vi "Begin.vi"(8 "error in":errorcluster) -> (0 "error out":errorcluster)   [LabVIEW 2020]
doc: "Called before other user functions, this VI is expected to open initial I/O refnums, load in file data, and do all program initialization. Notice that the <B>error out</B> terminal is simply used for data flow. Wiring it to other structures or subVIs ensures that this VI runs first."
uses:
  <vilib>/Rock Robotics/WPI/DriverStation/WPI_DriverStationRobotMode2.ctl
  <vilib>/Rock Robotics/WPI/Joystick/WPI_JoystickDeviceEnum.ctl
  <vilib>/Rock Robotics/SystemInterfaces/i2clib/i2c_bus.ctl
  <vilib>/Rock Robotics/WPI/Solenoid/WPI_SolenoidChannel.ctl
  <vilib>/Rock Robotics/SystemInterfaces/DIO/FPGA_DIOChannel.ctl
  Robot Global Data.vi
  <vilib>/Rock Robotics/Network Tables/NT Write String Array.vi
  <vilib>/Rock Robotics/WPI/ThirdParty/Phoenix-LabVIEW/Motor Controller/Get/CTRE_Phoenix_MotorController_GetSelectedSensorData.vi
  <vilib>/Rock Robotics/WPI/Solenoid/WPI_SolenoidOpenDouble.vi
  <vilib>/Rock Robotics/WPI/Switch/WPI_SwitchOpenLimit.vi
  <vilib>/Rock Robotics/WPI/Switch/WPI_SwitchOpenCounting.vi
  <vilib>/Rock Robotics/WPI/ThirdParty/Phoenix-LabVIEW/Motor Controller/Get/CTRE_Phoenix_MotorController_IntegratedSensorData_TalonFX.vi
  GlobalAutonVariables.vi
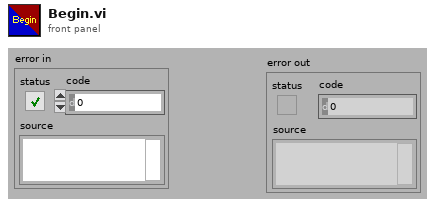
[diagram p1: front panel]
types:
  T1 = typedef "FPGA_DIOChannel.ctl" = enum8{"DIO 0", "DIO 1", "DIO 2", "DIO 3", "DIO 4", "DIO 5", "DIO 6", "DIO 7", "DIO 8", "DIO 9", "DIO MXP 0", "DIO MXP 1", "DIO MXP 2", "DIO MXP 3", "DIO MXP 4", "DIO MXP 5", "DIO MXP 6", "DIO MXP 7", "DIO MXP 8", "DIO MXP 9", "DIO MXP 10", "DIO MXP 11", "DIO MXP 12", "DIO MXP 13", "DIO MXP 14", "DIO MXP 15", "SPI Port CS1", "SPI Port CS2", "SPI Port CS3", "SPI Port MISO", "SPI Port MOSI", "Invalid"}
  T2 = typedef "WPI_SolenoidChannel.ctl" = enum8{"Solenoid 0", "Solenoid 1", "Solenoid 2", "Solenoid 3", "Solenoid 4", "Solenoid 5", "Solenoid 6", "Solenoid 7", "Solenoid 8", "Solenoid 9", "Solenoid 10", "Solenoid 11", "Solenoid 12", "Solenoid 13", "Solenoid 14", "Solenoid 15", "Invalid"}
  T3 = typedef "i2c_bus.ctl" = enum16{"I2C On-Board", "I2C MXP", "Invalid"}
  T4 = typedef "WPI_JoystickDeviceEnum.ctl" = enum16{"USB 0", "USB 1", "USB 2", "USB 3", "USB 4", "USB 5"}
  T5 = typedef "WPI_DriverStationRobotMode2.ctl" = enum16{"Autonomous Disabled", "Autonomous Enabled", "Teleop Disabled", "Teleop Enabled", "Disconnected", "Finish", "Test Disabled", "Test Enabled", "Emergency Stopped"}
  T6 = typedef "WPI_CompressorDevRef.ctl" = cluster{"DevStatus":errorcluster, "Pneumatics Control Module":u8}
  T7 = typedef "WPI_SolenoidDevRef.ctl" = cluster{"DevStatus":errorcluster, "Pneumatics Control Module":u8, "Forward Solenoid Channel":T2, "Reverse Solenoid Channel":T2}
  T8 = typedef "WPI_JoystickDevRef.ctl" = cluster{"Device":T4}
  T9 = typedef "WPI_MotorControlDeviceRef.ctl" = cluster{"DeviceStatus":errorcluster, "Type":T10, "PWM":cluster{"PWM Channel":T11, "DeadBand":T12}, "CAN":cluster{"Device Number":u8, "SetOutput VI Ref":variant, "GetOutput VI Ref":variant, "Enable VI Ref":variant, "Disable VI Ref":variant, "Data":variant}, "Invert":bool, "DIO PWM":cluster{"PWM \"Enable\" Channel":T11, "DIOChannel":T1, "PWM Rate":dbl}}
  T10 = typedef "WPI_MotorControlType.ctl" = enum16{"PWM", "CAN", "DIO PWM"}
  T11 = typedef "FPGA_DIOPWMChannel.ctl" = enum8{"PWM 0", "PWM 1", "PWM 2", "PWM 3", "PWM 4", "PWM 5", "PWM 6", "PWM 7", "PWM 8", "PWM 9", "PWM MXP 0", "PWM MXP 1", "PWM MXP 2", "PWM MXP 3", "PWM MXP 4", "PWM MXP 5", "PWM MXP 6", "PWM MXP 7", "PWM MXP 8", "PWM MXP 9", "Invalid"}
  T12 = typedef "WPI_PWMDeadband.ctl" = cluster{"Name":string, "maxPositivePwm":i32, "minPositivePwm":i32, "centerPwm":i32, "maxNegativePwm":i32, "minNegativePwm":i32, "angularRange":u16}
  T13 = typedef "Color Sensor V3 DevRef.ctl" = cluster{"I2CDevRef":T14}
  T14 = typedef "WPI_I2CDevRef.ctl" = cluster{"DevStatus":errorcluster, "Device Address":u8, "Handle":i32, "I2C Bus":T3}
  T15 = typedef "CTRE_PigeonIMU_DeviceRef.ctl" = cluster{"DeviceStatus":errorcluster, "Device Number":u8, "Type":T16, "Device ID":u32, "Handle":u64, "UsageFrame":u32, "Library Path":path}
  T16 = typedef "CTRE_PigeonIMU_ConnectionType.ctl" = u32
  T17 = typedef "CTRE_Phoenix_CANcoder_DeviceRef.ctl" = cluster{"DeviceStatus":errorcluster, "Device Number":u8, "Handle":u64, "UsageFrame":u32, "Library Path":path}
  T18 = typedef "WPI_SwitchDevRef.ctl" = cluster{"DevStatus":errorcluster, "DIO Channel":T1, "CntIndex":T19, "Normally Closed":bool}
  T19 = typedef "FPGA_CounterCtrSystemIndex.ctl" = enum8{"Ctr 0", "Ctr 1", "Ctr 2", "Ctr 3", "Ctr 4", "Ctr 5", "Ctr 6", "Ctr 7", "Invalid"}
  T20 = enum16{"open", "replace", "create", "open or create", "replace or create", "replace or create with confirmation"}
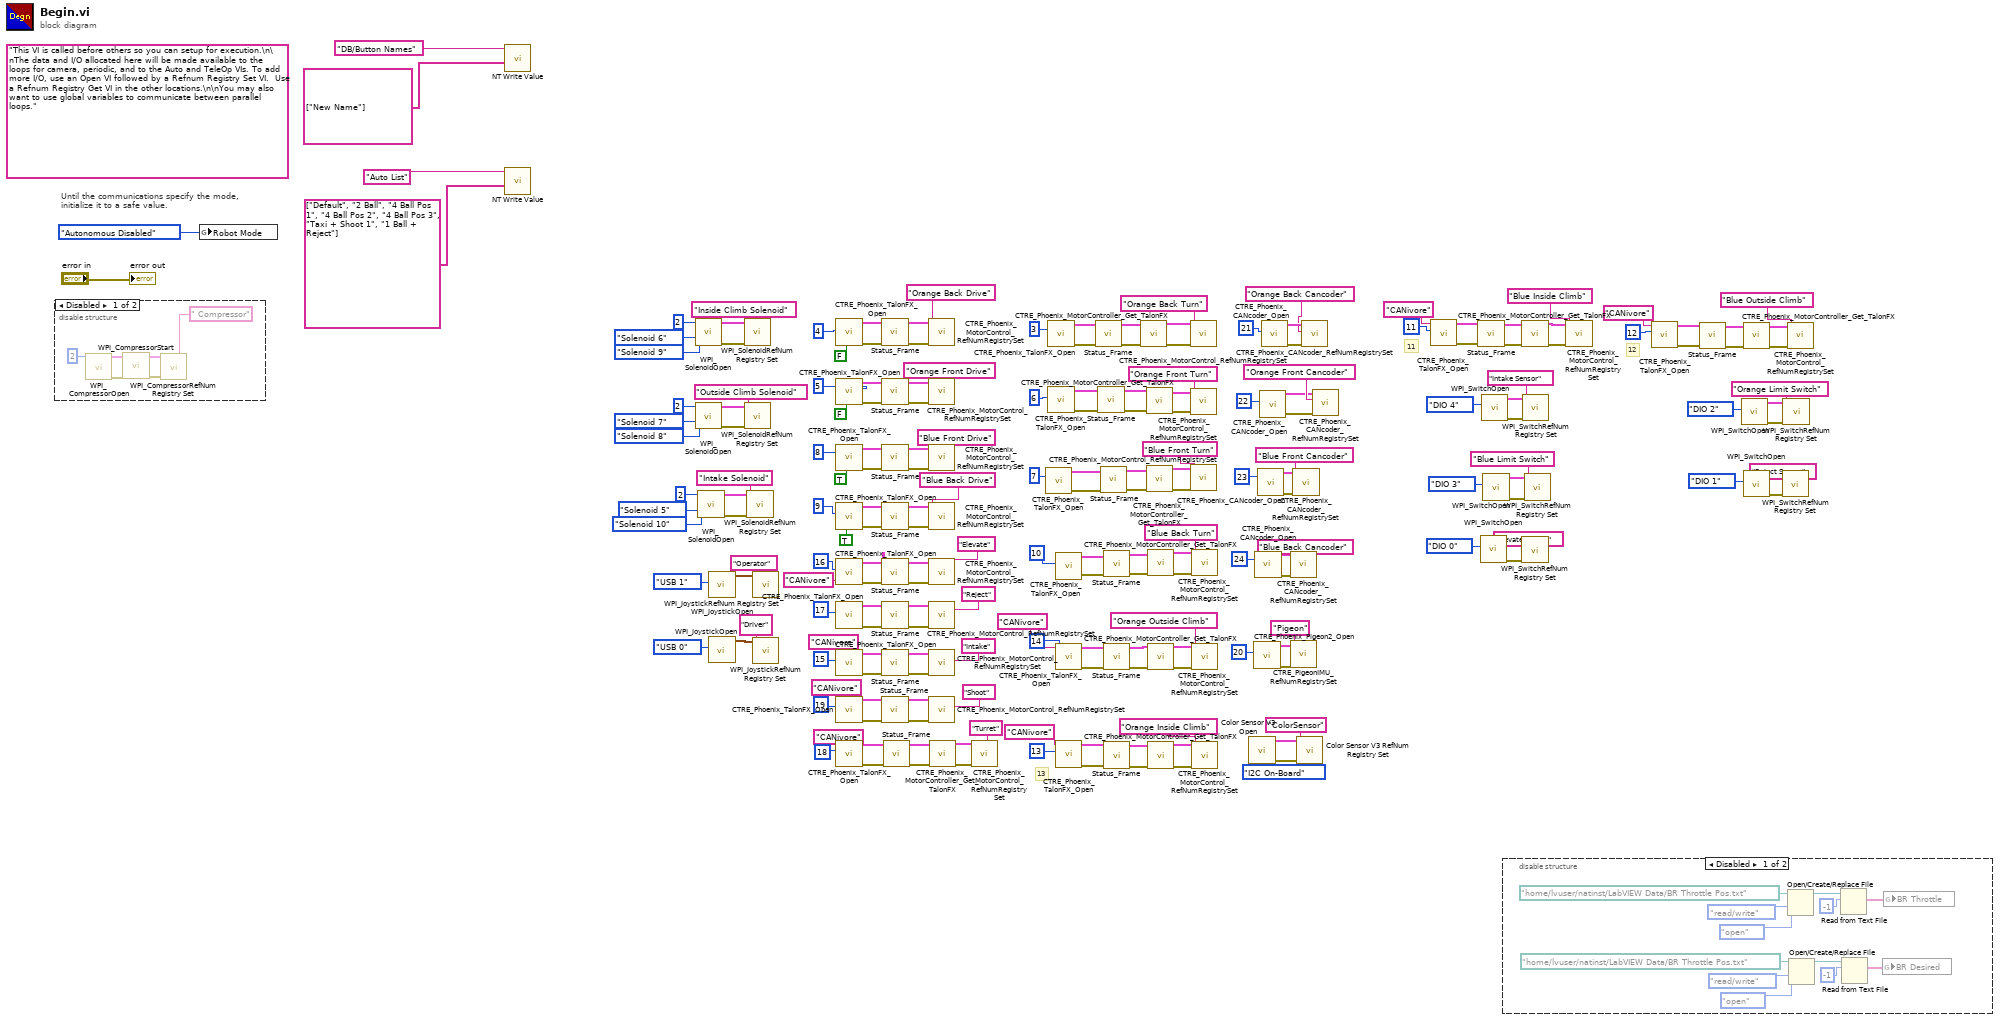
[diagram p0: block diagram]
diagram:
  (unwired) "This VI is called before others so you can setup for execution.\n\nThe data and I/O allocated here will be made available to the loops for camera, periodic, and to the Auto and TeleOp VIs. To add more I/O, use an Open VI followed by a Refnum Registry Set VI.  Use a Refnum Registry Get VI in the other locations.\n\nYou may also want to use global variables to communicate between parallel loops."
  # "13"
  # "12"
  # "11"
  # "Until the communications specify the mode,\ninitialize it to a safe value."
  n1 = disable-structure shown="Disabled" {
    frame Disabled {
      n2 = call <vilib>:"WPI_CompressorOpen.vi"("Pneumatics device (def)"=u8 2) -> ("CompressorDevRef"=w211:T6, "error out"=w212:errorcluster)  [unwired: 13 in]
      n3 = call <vilib>:"WPI_CompressorStart.vi"("error in (no error)"=w212, "CompressorDevRef"=w211) -> ("error out"=w210:errorcluster, "CompressorDevRef"=w209:T6)  [unwired: 8 in]
      n4 = call <vilib>:"WPI_CompressorRefNum Registry Set.vi"("error in (no error)"=w210, "refnum name"=" Compressor", "CompressorDevRef"=w209) -> ()  [unwired: 7 in, 2 out]
    }
    frame Enabled {
    }
  }
  n5 = global write "Robot Global Data.vi" "Robot Mode"(WPI_DriverStationRobotMode2."Autonomous Disabled" ("Robot Mode")) -> ()
  n6 = call-poly <vilib>:"NT Write Value.vi"("String Array"=string[] ["New Name"], "Name"="DB/Button Names") -> ()  [unwired: 9 in, 1 out]
  n7 = call-poly <vilib>:"NT Write Value.vi"("String Array"=string[] ["Default", "2 Ball", "4 Ball Pos 1", "4 Ball Pos 2", "4 Ball Pos 3", "Taxi + Shoot 1", "1 Ball + Reject"], "Name"="Auto List") -> ()  [unwired: 9 in, 1 out]
  n8 = call-poly <vilib>:"WPI_SolenoidOpen.vi"("Reverse Solenoid Channel"=WPI_SolenoidChannel."Solenoid 9", "Forward Solenoid Channel"=WPI_SolenoidChannel."Solenoid 6", "Pneumatics Device (def)"=u8 2) -> ("error out"=w155:errorcluster, "SolenoidDevRef"=w154:T7)  [unwired: 7 in]
  n9 = call-poly <vilib>:"WPI_SolenoidOpen.vi"("Reverse Solenoid Channel"=WPI_SolenoidChannel."Solenoid 8", "Forward Solenoid Channel"=WPI_SolenoidChannel."Solenoid 7", "Pneumatics Device (def)"=u8 2) -> ("error out"=w152:errorcluster, "SolenoidDevRef"=w151:T7)  [unwired: 7 in]
  n10 = call-poly <vilib>:"WPI_SolenoidOpen.vi"("Reverse Solenoid Channel"=WPI_SolenoidChannel."Solenoid 10", "Forward Solenoid Channel"=WPI_SolenoidChannel."Solenoid 5", "Pneumatics Device (def)"=u8 2) -> ("error out"=w149:errorcluster, "SolenoidDevRef"=w148:T7)  [unwired: 7 in]
  n11 = call <vilib>:"WPI_JoystickOpen.vi"("JoystickDevice"=WPI_JoystickDeviceEnum."USB 1") -> ("JoystickDevRef"=w196:T8)  [unwired: 10 in]
  n12 = call <vilib>:"WPI_JoystickOpen.vi"("JoystickDevice"=WPI_JoystickDeviceEnum."USB 0") -> ("JoystickDevRef"=w204:T8)  [unwired: 10 in]
  n13 = call <vilib>:"WPI_SolenoidRefNum Registry Set.vi"("error in (no error)"=w155, "refnum name"="Inside Climb Solenoid", "SolenoidDevRef"=w154) -> ()  [unwired: 7 in, 2 out]
  n14 = call <vilib>:"WPI_SolenoidRefNum Registry Set.vi"("error in (no error)"=w152, "refnum name"="Outside Climb Solenoid", "SolenoidDevRef"=w151) -> ()  [unwired: 7 in, 2 out]
  n15 = call <vilib>:"WPI_SolenoidRefNum Registry Set.vi"("error in (no error)"=w149, "refnum name"="Intake Solenoid", "SolenoidDevRef"=w148) -> ()  [unwired: 7 in, 2 out]
  n16 = call <vilib>:"WPI_JoystickRefNum Registry Set.vi"("refnum name"="Operator", "JoystickDevRef"=w196) -> ()  [unwired: 8 in, 2 out]
  n17 = call <vilib>:"WPI_JoystickRefNum Registry Set.vi"("refnum name"="Driver", "JoystickDevRef"=w204) -> ()  [unwired: 8 in, 2 out]
  n18 = call <vilib>:"CTRE_Phoenix_TalonFX_Open.vi"("Invert"=FALSE, "Device Number"=u8 4) -> ("error out"=w75:errorcluster, "PhoenixMotorControlDevRef"=w76:T9)  [unwired: 8 in]
  n19 = call <vilib>:"CTRE_Phoenix_TalonFX_Open.vi"("Invert"=FALSE, "Device Number"=u8 5) -> ("error out"=w68:errorcluster, "PhoenixMotorControlDevRef"=w67:T9)  [unwired: 8 in]
  n20 = call <vilib>:"CTRE_Phoenix_TalonFX_Open.vi"("Invert"=TRUE, "Device Number"=u8 8) -> ("error out"=w72:errorcluster, "PhoenixMotorControlDevRef"=w69:T9)  [unwired: 8 in]
  n21 = call <vilib>:"CTRE_Phoenix_TalonFX_Open.vi"("Invert"=TRUE, "Device Number"=u8 9) -> ("error out"=w61:errorcluster, "PhoenixMotorControlDevRef"=w64:T9)  [unwired: 8 in]
  n22 = call <vilib>:"CTRE_Phoenix_TalonFX_Open.vi"("Device Number"=u8 16, "CAN Bus"="CANivore") -> ("error out"=w57:errorcluster, "PhoenixMotorControlDevRef"=w60:T9)  [unwired: 8 in]
  n23 = call <vilib>:"CTRE_Phoenix_TalonFX_Open.vi"("Device Number"=u8 17) -> ("error out"=w53:errorcluster, "PhoenixMotorControlDevRef"=w56:T9)  [unwired: 9 in]
  n24 = call <vilib>:"CTRE_Phoenix_TalonFX_Open.vi"("Device Number"=u8 15, "CAN Bus"="CANivore") -> ("error out"=w49:errorcluster, "PhoenixMotorControlDevRef"=w52:T9)  [unwired: 8 in]
  n25 = call <vilib>:"CTRE_Phoenix_TalonFX_Open.vi"("Device Number"=u8 19, "CAN Bus"="CANivore") -> ("error out"=w45:errorcluster, "PhoenixMotorControlDevRef"=w48:T9)  [unwired: 8 in]
  n26 = call <vilib>:"CTRE_Phoenix_TalonFX_Open.vi"("Device Number"=u8 18, "CAN Bus"="CANivore") -> ("error out"=w42:errorcluster, "PhoenixMotorControlDevRef"=w43:T9)  [unwired: 8 in]
  n27 = call "Status_Frame.vi"("error in (no error)"=w75, "Motor Control DevRef"=w76) -> ("error out"=w74:errorcluster, "PhoenixMotorControlDevRef"=w73:T9)  [unwired: 8 in]
  n28 = call "Status_Frame.vi"("error in (no error)"=w68, "Motor Control DevRef"=w67) -> ("error out"=w65:errorcluster, "PhoenixMotorControlDevRef"=w66:T9)  [unwired: 8 in]
  n29 = call "Status_Frame.vi"("error in (no error)"=w72, "Motor Control DevRef"=w69) -> ("error out"=w71:errorcluster, "PhoenixMotorControlDevRef"=w70:T9)  [unwired: 8 in]
  n30 = call "Status_Frame.vi"("error in (no error)"=w61, "Motor Control DevRef"=w64) -> ("error out"=w62:errorcluster, "PhoenixMotorControlDevRef"=w63:T9)  [unwired: 8 in]
  n31 = call "Status_Frame.vi"("error in (no error)"=w57, "Motor Control DevRef"=w60) -> ("error out"=w58:errorcluster, "PhoenixMotorControlDevRef"=w59:T9)  [unwired: 8 in]
  n32 = call "Status_Frame.vi"("error in (no error)"=w53, "Motor Control DevRef"=w56) -> ("error out"=w54:errorcluster, "PhoenixMotorControlDevRef"=w55:T9)  [unwired: 8 in]
  n33 = call "Status_Frame.vi"("error in (no error)"=w49, "Motor Control DevRef"=w52) -> ("error out"=w50:errorcluster, "PhoenixMotorControlDevRef"=w51:T9)  [unwired: 8 in]
  n34 = call "Status_Frame.vi"("error in (no error)"=w45, "Motor Control DevRef"=w48) -> ("error out"=w46:errorcluster, "PhoenixMotorControlDevRef"=w47:T9)  [unwired: 8 in]
  n35 = call "Status_Frame.vi"("error in (no error)"=w42, "Motor Control DevRef"=w43) -> ("error out"=w3:errorcluster, "PhoenixMotorControlDevRef"=w4:T9)  [unwired: 8 in]
  n36 = call <vilib>:"CTRE_Phoenix_MotorControl_RefNumRegistrySet.vi"("error in (no error)"=w74, "refnum name"="Orange Back Drive", "PhoenixMotorControlDevRef"=w73) -> ()  [unwired: 7 in, 2 out]
  n37 = call <vilib>:"CTRE_Phoenix_MotorControl_RefNumRegistrySet.vi"("error in (no error)"=w65, "refnum name"="Orange Front Drive", "PhoenixMotorControlDevRef"=w66) -> ()  [unwired: 7 in, 2 out]
  n38 = call <vilib>:"CTRE_Phoenix_MotorControl_RefNumRegistrySet.vi"("error in (no error)"=w71, "refnum name"="Blue Front Drive", "PhoenixMotorControlDevRef"=w70) -> ()  [unwired: 7 in, 2 out]
  n39 = call <vilib>:"CTRE_Phoenix_MotorControl_RefNumRegistrySet.vi"("error in (no error)"=w62, "refnum name"="Blue Back Drive", "PhoenixMotorControlDevRef"=w63) -> ()  [unwired: 7 in, 2 out]
  n40 = call <vilib>:"CTRE_Phoenix_MotorControl_RefNumRegistrySet.vi"("error in (no error)"=w58, "refnum name"="Elevate", "PhoenixMotorControlDevRef"=w59) -> ()  [unwired: 7 in, 2 out]
  n41 = call <vilib>:"CTRE_Phoenix_MotorControl_RefNumRegistrySet.vi"("error in (no error)"=w54, "refnum name"="Reject", "PhoenixMotorControlDevRef"=w55) -> ()  [unwired: 7 in, 2 out]
  n42 = call <vilib>:"CTRE_Phoenix_MotorControl_RefNumRegistrySet.vi"("error in (no error)"=w50, "refnum name"="Intake", "PhoenixMotorControlDevRef"=w51) -> ()  [unwired: 7 in, 2 out]
  n43 = call <vilib>:"CTRE_Phoenix_MotorControl_RefNumRegistrySet.vi"("error in (no error)"=w46, "refnum name"="Shoot", "PhoenixMotorControlDevRef"=w47) -> ()  [unwired: 7 in, 2 out]
  n44 = call-poly <vilib>:"CTRE_Phoenix_MotorController_Get_TalonFX.vi"("PhoenixMotorControlDevRef"=w4, "error in"=w3) -> ("PhoenixMotorControlDevRef"=w1:T9, "error out"=w2:errorcluster)  [unwired: 9 in, 3 out]
  n45 = call <vilib>:"CTRE_Phoenix_MotorControl_RefNumRegistrySet.vi"("error in (no error)"=w2, "refnum name"="Turret", "PhoenixMotorControlDevRef"=w1) -> ()  [unwired: 7 in, 2 out]
  n46 = call <vilib>:"CTRE_Phoenix_TalonFX_Open.vi"("Device Number"=u8 7) -> ("error out"=w30:errorcluster, "PhoenixMotorControlDevRef"=w33:T9)  [unwired: 9 in]
  n47 = call <vilib>:"CTRE_Phoenix_TalonFX_Open.vi"("Device Number"=u8 3) -> ("error out"=w38:errorcluster, "PhoenixMotorControlDevRef"=w41:T9)  [unwired: 9 in]
  n48 = call <vilib>:"CTRE_Phoenix_TalonFX_Open.vi"("Device Number"=u8 6) -> ("error out"=w34:errorcluster, "PhoenixMotorControlDevRef"=w37:T9)  [unwired: 9 in]
  n49 = call <vilib>:"CTRE_Phoenix_TalonFX_Open.vi"("Device Number"=u8 10) -> ("error out"=w26:errorcluster, "PhoenixMotorControlDevRef"=w27:T9)  [unwired: 9 in]
  n50 = call <vilib>:"CTRE_Phoenix_TalonFX_Open.vi"("Device Number"=u8 14, "CAN Bus"="CANivore") -> ("error out"=w16:errorcluster, "PhoenixMotorControlDevRef"=w17:T9)  [unwired: 8 in]
  n51 = call <vilib>:"CTRE_Phoenix_TalonFX_Open.vi"("Device Number"=u8 13, "CAN Bus"="CANivore") -> ("error out"=w14:errorcluster, "PhoenixMotorControlDevRef"=w15:T9)  [unwired: 8 in]
  n52 = call "Status_Frame.vi"("error in (no error)"=w38, "Motor Control DevRef"=w41) -> ("error out"=w39:errorcluster, "PhoenixMotorControlDevRef"=w40:T9)  [unwired: 8 in]
  n53 = call "Status_Frame.vi"("error in (no error)"=w34, "Motor Control DevRef"=w37) -> ("error out"=w35:errorcluster, "PhoenixMotorControlDevRef"=w36:T9)  [unwired: 8 in]
  n54 = call "Status_Frame.vi"("error in (no error)"=w30, "Motor Control DevRef"=w33) -> ("error out"=w31:errorcluster, "PhoenixMotorControlDevRef"=w32:T9)  [unwired: 8 in]
  n55 = call "Status_Frame.vi"("error in (no error)"=w26, "Motor Control DevRef"=w27) -> ("error out"=w28:errorcluster, "PhoenixMotorControlDevRef"=w29:T9)  [unwired: 8 in]
  n56 = call "Status_Frame.vi"("error in (no error)"=w16, "Motor Control DevRef"=w17) -> ("error out"=w24:errorcluster, "PhoenixMotorControlDevRef"=w25:T9)  [unwired: 8 in]
  n57 = call "Status_Frame.vi"("error in (no error)"=w14, "Motor Control DevRef"=w15) -> ("error out"=w22:errorcluster, "PhoenixMotorControlDevRef"=w23:T9)  [unwired: 8 in]
  n58 = call-poly <vilib>:"CTRE_Phoenix_MotorController_Get_TalonFX.vi"("PhoenixMotorControlDevRef"=w40, "error in"=w39) -> ("PhoenixMotorControlDevRef"=w92:T9, "error out"=w194:errorcluster)  [unwired: 10 in, 2 out]
  n59 = call-poly <vilib>:"CTRE_Phoenix_MotorController_Get_TalonFX.vi"("PhoenixMotorControlDevRef"=w36, "error in"=w35) -> ("PhoenixMotorControlDevRef"=w187:T9, "error out"=w188:errorcluster)  [unwired: 10 in, 2 out]
  n60 = call-poly <vilib>:"CTRE_Phoenix_MotorController_Get_TalonFX.vi"("PhoenixMotorControlDevRef"=w32, "error in"=w31) -> ("PhoenixMotorControlDevRef"=w98:T9, "error out"=w93:errorcluster)  [unwired: 10 in, 2 out]
  n61 = call-poly <vilib>:"CTRE_Phoenix_MotorController_Get_TalonFX.vi"("PhoenixMotorControlDevRef"=w29, "error in"=w28) -> ("PhoenixMotorControlDevRef"=w94:T9, "error out"=w175:errorcluster)  [unwired: 10 in, 2 out]
  n62 = call-poly <vilib>:"CTRE_Phoenix_MotorController_Get_TalonFX.vi"("PhoenixMotorControlDevRef"=w25, "error in"=w24) -> ("PhoenixMotorControlDevRef"=w95:T9, "error out"=w112:errorcluster)  [unwired: 10 in, 2 out]
  n63 = call-poly <vilib>:"CTRE_Phoenix_MotorController_Get_TalonFX.vi"("PhoenixMotorControlDevRef"=w23, "error in"=w22) -> ("PhoenixMotorControlDevRef"=w97:T9, "error out"=w109:errorcluster)  [unwired: 10 in, 2 out]
  n64 = call <vilib>:"CTRE_Phoenix_MotorControl_RefNumRegistrySet.vi"("error in (no error)"=w194, "refnum name"="Orange Back Turn", "PhoenixMotorControlDevRef"=w92) -> ()  [unwired: 7 in, 2 out]
  n65 = call <vilib>:"CTRE_Phoenix_MotorControl_RefNumRegistrySet.vi"("error in (no error)"=w188, "refnum name"="Orange Front Turn", "PhoenixMotorControlDevRef"=w187) -> ()  [unwired: 7 in, 2 out]
  n66 = call <vilib>:"CTRE_Phoenix_MotorControl_RefNumRegistrySet.vi"("error in (no error)"=w93, "refnum name"="Blue Front Turn", "PhoenixMotorControlDevRef"=w98) -> ()  [unwired: 7 in, 2 out]
  n67 = call <vilib>:"CTRE_Phoenix_MotorControl_RefNumRegistrySet.vi"("error in (no error)"=w175, "refnum name"="Blue Back Turn", "PhoenixMotorControlDevRef"=w94) -> ()  [unwired: 7 in, 2 out]
  n68 = call <vilib>:"CTRE_Phoenix_MotorControl_RefNumRegistrySet.vi"("error in (no error)"=w112, "refnum name"="Orange Outside Climb", "PhoenixMotorControlDevRef"=w95) -> ()  [unwired: 7 in, 2 out]
  n69 = call <vilib>:"CTRE_Phoenix_MotorControl_RefNumRegistrySet.vi"("error in (no error)"=w109, "refnum name"="Orange Inside Climb", "PhoenixMotorControlDevRef"=w97) -> ()  [unwired: 7 in, 2 out]
  n70 = call <vilib>:"Color Sensor V3 Open.vi"("I2C Bus"=i2c_bus."I2C On-Board") -> ("error out"=w159:errorcluster, "ColorSensorDevRef"=w158:T13)  [unwired: 9 in]
  n71 = call <vilib>:"CTRE_Phoenix_Pigeon2_Open.vi"("Device Number"=u8 20) -> ("error out"=w5:errorcluster, "PigeonIMUDevRef"=w6:T15)  [unwired: 9 in]
  n72 = call <vilib>:"CTRE_Phoenix_CANcoder_Open.vi"("Device Number"=u8 24) -> ("error out"=w87:errorcluster, "CTRE_CANcoder_DeviceRef"=w88:T17)  [unwired: 9 in]
  n73 = call <vilib>:"CTRE_Phoenix_CANcoder_Open.vi"("Device Number"=u8 23) -> ("error out"=w89:errorcluster, "CTRE_CANcoder_DeviceRef"=w90:T17)  [unwired: 9 in]
  n74 = call <vilib>:"CTRE_Phoenix_CANcoder_Open.vi"("Device Number"=u8 22) -> ("error out"=w86:errorcluster, "CTRE_CANcoder_DeviceRef"=w85:T17)  [unwired: 9 in]
  n75 = call <vilib>:"CTRE_Phoenix_CANcoder_Open.vi"("Device Number"=u8 21) -> ("error out"=w8:errorcluster, "CTRE_CANcoder_DeviceRef"=w9:T17)  [unwired: 9 in]
  n76 = call <vilib>:"CTRE_Phoenix_CANcoder_RefNumRegistrySet.vi"("error in (no error)"=w87, "refnum name"="Blue Back Cancoder", "CTRE_CANcoder_DeviceRef"=w88) -> ()  [unwired: 7 in, 2 out]
  n77 = call <vilib>:"CTRE_PigeonIMU_RefNumRegistrySet.vi"("error in (no error)"=w5, "refnum name"="Pigeon", "PigeonIMUDevRef"=w6) -> ()  [unwired: 7 in, 2 out]
  n78 = call <vilib>:"CTRE_Phoenix_CANcoder_RefNumRegistrySet.vi"("error in (no error)"=w89, "refnum name"="Blue Front Cancoder", "CTRE_CANcoder_DeviceRef"=w90) -> ()  [unwired: 7 in, 2 out]
  n79 = call <vilib>:"Color Sensor V3 RefNum Registry Set.vi"("error in (no error)"=w159, "refnum name"="ColorSensor", "ColorSensorDevRef"=w158) -> ()  [unwired: 7 in, 2 out]
  n80 = call <vilib>:"CTRE_Phoenix_CANcoder_RefNumRegistrySet.vi"("error in (no error)"=w8, "refnum name"="Orange Back Cancoder", "CTRE_CANcoder_DeviceRef"=w9) -> ()  [unwired: 7 in, 2 out]
  n81 = call <vilib>:"CTRE_Phoenix_CANcoder_RefNumRegistrySet.vi"("error in (no error)"=w86, "refnum name"="Orange Front Cancoder", "CTRE_CANcoder_DeviceRef"=w85) -> ()  [unwired: 7 in, 2 out]
  n82 = call <vilib>:"CTRE_Phoenix_TalonFX_Open.vi"("Device Number"=u8 11, "CAN Bus"="CANivore") -> ("error out"=w10:errorcluster, "PhoenixMotorControlDevRef"=w11:T9)  [unwired: 8 in]
  n83 = call "Status_Frame.vi"("error in (no error)"=w10, "Motor Control DevRef"=w11) -> ("error out"=w18:errorcluster, "PhoenixMotorControlDevRef"=w19:T9)  [unwired: 8 in]
  n84 = call-poly <vilib>:"WPI_SwitchOpen.vi"("DIO Channel"=FPGA_DIOChannel."DIO 0") -> ("error out"=w137:errorcluster, "SwitchDevRef"=w136:T18)  [unwired: 9 in]
  n85 = call-poly <vilib>:"WPI_SwitchOpen.vi"("DIO Channel"=FPGA_DIOChannel."DIO 4") -> ("error out"=w116:errorcluster, "SwitchDevRef"=w115:T18)  [unwired: 9 in]
  n86 = call-poly <vilib>:"WPI_SwitchOpen.vi"("DIO Channel"=FPGA_DIOChannel."DIO 3") -> ("error out"=w120:errorcluster, "SwitchDevRef"=w119:T18)  [unwired: 9 in]
  n87 = disable-structure shown="Disabled" {
    frame Disabled {
      n88 = Open/Create/Replace File(file path (use dialog)=path "/home/lvuser/natinst/LabVIEW Data/BR Throttle Pos.txt", operation (0:open)=T20."open", access (0:read/write)=enum16{"read/write", "read-only", "write-only"}."read/write") -> (refnum out=w221:refnum<file>)  [unwired: 3 in, 2 out]
      n89 = Open/Create/Replace File(file path (use dialog)=path "/home/lvuser/natinst/LabVIEW Data/BR Throttle Pos.txt", operation (0:open)=T20."open", access (0:read/write)=enum16{"read/write", "read-only", "write-only"}."read/write") -> (refnum out=w216:refnum<file>)  [unwired: 3 in, 2 out]
      n90 = Read from Text File(file (use dialog)=w221, count=-1) -> (text=w214:string[])  [unwired: 2 in, 3 out]
      n91 = Read from Text File(file (use dialog)=w216, count=-1) -> (text=w213:string[])  [unwired: 2 in, 3 out]
      n92 = global write "GlobalAutonVariables.vi" "BR Desired"(w213) -> ()
      n93 = global write "GlobalAutonVariables.vi" "BR Throttle"(w214) -> ()
    }
    frame Enabled {
    }
  }
  n94 = call-poly <vilib>:"CTRE_Phoenix_MotorController_Get_TalonFX.vi"("PhoenixMotorControlDevRef"=w19, "error in"=w18) -> ("PhoenixMotorControlDevRef"=w101:T9, "error out"=w102:errorcluster)  [unwired: 10 in, 2 out]
  n95 = call <vilib>:"WPI_SwitchRefNum Registry Set.vi"("error in (no error)"=w137, "refnum name"="Elevate Sensor", "SwitchDevRef"=w136) -> ()  [unwired: 7 in, 2 out]
  n96 = call <vilib>:"WPI_SwitchRefNum Registry Set.vi"("error in (no error)"=w116, "refnum name"="Intake Sensor", "SwitchDevRef"=w115) -> ()  [unwired: 7 in, 2 out]
  n97 = call <vilib>:"WPI_SwitchRefNum Registry Set.vi"("error in (no error)"=w120, "refnum name"="Blue Limit Switch", "SwitchDevRef"=w119) -> ()  [unwired: 7 in, 2 out]
  n98 = call <vilib>:"CTRE_Phoenix_MotorControl_RefNumRegistrySet.vi"("error in (no error)"=w102, "refnum name"="Blue Inside Climb", "PhoenixMotorControlDevRef"=w101) -> ()  [unwired: 7 in, 2 out]
  n99 = call <vilib>:"CTRE_Phoenix_TalonFX_Open.vi"("Device Number"=u8 12, "CAN Bus"="CANivore") -> ("error out"=w12:errorcluster, "PhoenixMotorControlDevRef"=w13:T9)  [unwired: 8 in]
  n100 = call "Status_Frame.vi"("error in (no error)"=w12, "Motor Control DevRef"=w13) -> ("error out"=w20:errorcluster, "PhoenixMotorControlDevRef"=w21:T9)  [unwired: 8 in]
  n101 = call-poly <vilib>:"WPI_SwitchOpen.vi"("DIO Channel"=FPGA_DIOChannel."DIO 2") -> ("error out"=w124:errorcluster, "SwitchDevRef"=w123:T18)  [unwired: 9 in]
  n102 = call-poly <vilib>:"CTRE_Phoenix_MotorController_Get_TalonFX.vi"("PhoenixMotorControlDevRef"=w21, "error in"=w20) -> ("PhoenixMotorControlDevRef"=w105:T9, "error out"=w106:errorcluster)  [unwired: 10 in, 2 out]
  n103 = call-poly <vilib>:"WPI_SwitchOpen.vi"("DIO Channel"=FPGA_DIOChannel."DIO 1") -> ("error out"=w133:errorcluster, "SwitchDevRef"=w132:T18)  [unwired: 9 in]
  n104 = call <vilib>:"WPI_SwitchRefNum Registry Set.vi"("error in (no error)"=w133, "refnum name"="Reject Sensor", "SwitchDevRef"=w132) -> ()  [unwired: 7 in, 2 out]
  n105 = call <vilib>:"WPI_SwitchRefNum Registry Set.vi"("error in (no error)"=w124, "refnum name"="Orange Limit Switch", "SwitchDevRef"=w123) -> ()  [unwired: 7 in, 2 out]
  n106 = call <vilib>:"CTRE_Phoenix_MotorControl_RefNumRegistrySet.vi"("error in (no error)"=w106, "refnum name"="Blue Outside Climb", "PhoenixMotorControlDevRef"=w105) -> ()  [unwired: 7 in, 2 out]
  "error out" <- "error in"
